vi "Create.vi"(8 "error in (no error)":errorcluster, 10 "UART #":T1=-1) -> (0 "error out":errorcluster, 3 "UART out":refnum<class "UART.lvclass">)   [LabVIEW 2020, in "CTI.lvlib" / "UART.lvclass"]
uses:
  UART.lvclass
  UART Number.ctl
  UART.lvclass/UART.ctl
  CTI.lvlib
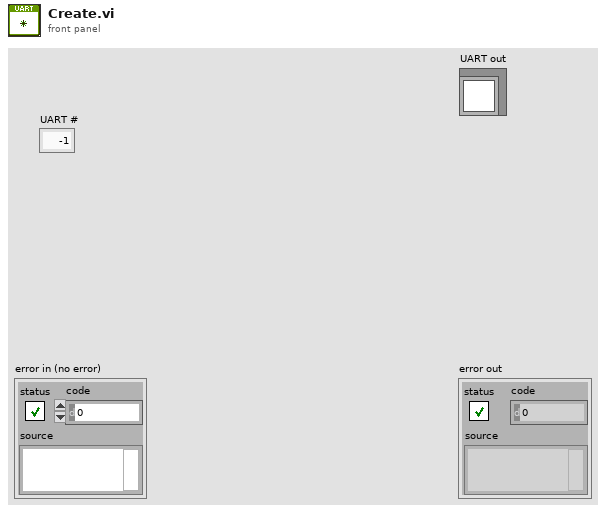
[diagram p1: front panel]
types:
  T1 = typedef "CTI.lvlib/UART Number.ctl" = i8
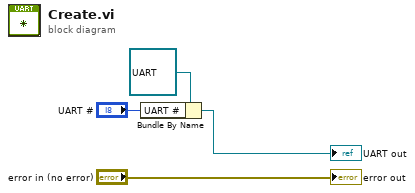
[diagram p0: block diagram]
diagram:
  n1 = Bundle By Name(cluster=refnum<class "UART.lvclass"> refnum ("UART in"), "UART #"="UART #") -> (→"UART out":refnum<class "UART.lvclass">)
  "error out" <- "error in (no error)"
